vi "Get VS Amplitude From String.vi"(10 "index":i32, 11 "text":string) -> (1 "function return":u32, 2 "index out":i32, 3 "text out":string)   [LabVIEW 2018, in "Copy of Andor SDK.lvlib"]
doc: "EXPNETTYPE unsigned int WINAPI GetVSAmplitudeFromString(char * text, int * index);"
uses:
  Copy of Andor SDK.lvlib
  <userlib>/Andor SDK/ATMCD32D.dll
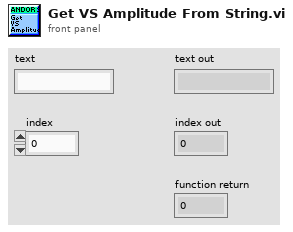
[diagram p1: front panel]
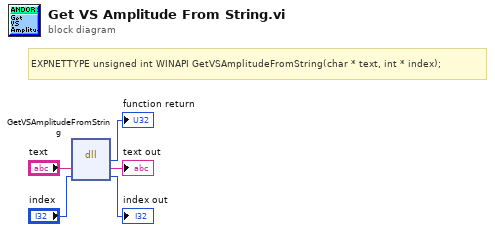
[diagram p0: block diagram]
diagram:
  # "EXPNETTYPE unsigned int WINAPI GetVSAmplitudeFromString(char * text, int * index);"
  n1 = dll-call lib="C:/Program Files (x86)/National Instruments/LabVIEW 2018/user.lib/Andor SDK/ATMCD32D.*" fn="GetVSAmplitudeFromString"("text"="text", "index"="index") -> (→"function return":u32, "text"=→"text out":string, "index"=→"index out":i32)  [unwired: 3 in, 2 out]
